vi "New Dashboard.vi"() -> ()   [LabVIEW 2015]
uses:
  <vilib>/Rock Robotics/Network Tables/NT Read Number.vi
  <vilib>/Rock Robotics/Network Tables/NT Read Numeric Array.vi
panel:
  out "MotorChart L":T1(graph)
  out "MotorSliders L":T2 {"MotorSlide4 2" scale=0.0..14.0 scale format="%#_2e"; "MotorSlide2" scale=-1.0..1.0 scale format="%#_2e"; "MotorSlide1" scale=-1.0..1.0 scale format="%#_2e"}
  out "MotorChart R":cluster{"Numeric":dbl, "Numeric":dbl}(graph)
  out "MotorSliders R":cluster{"MotorSlide1":dbl, "MotorSlide2":dbl} {"MotorSlide2" scale=-1.0..1.0 scale format="%#_2e"; "MotorSlide1" scale=-1.0..1.0 scale format="%#_2e"}
  out "JS1 Graph":cluster{"X":dbl, "Y":dbl}[](graph)
  out "JS1 Z":dbl(slide) scale=-1.0..1.0 scale format="%#_2e"
  out "JS1 Buttons":T3
  out "Gyro":dbl(knob) scale=0.0..360.0
  out "JS2 Graph":cluster{"X":dbl, "Y":dbl}[](graph)
  out "JS2 Z":dbl(slide) scale=-1.0..1.0 scale format="%#_2e"
  out "JS2 Buttons":T3
  out "Camera IP":string
  in  "TCP":refnum<k5>
  out "Mode":T4(ring)=enum."Auto Disabled"
  in  "Vision":u16(ring) items=["Camera Off", "USB Camera SW", "USB Camera HW", "IP Camera"]
  in  "Rec Mode":enum32{"Stop", "Record", "Playback"}(radio)
  out "Air Pressure":dbl(knob) scale=0.0..150.0
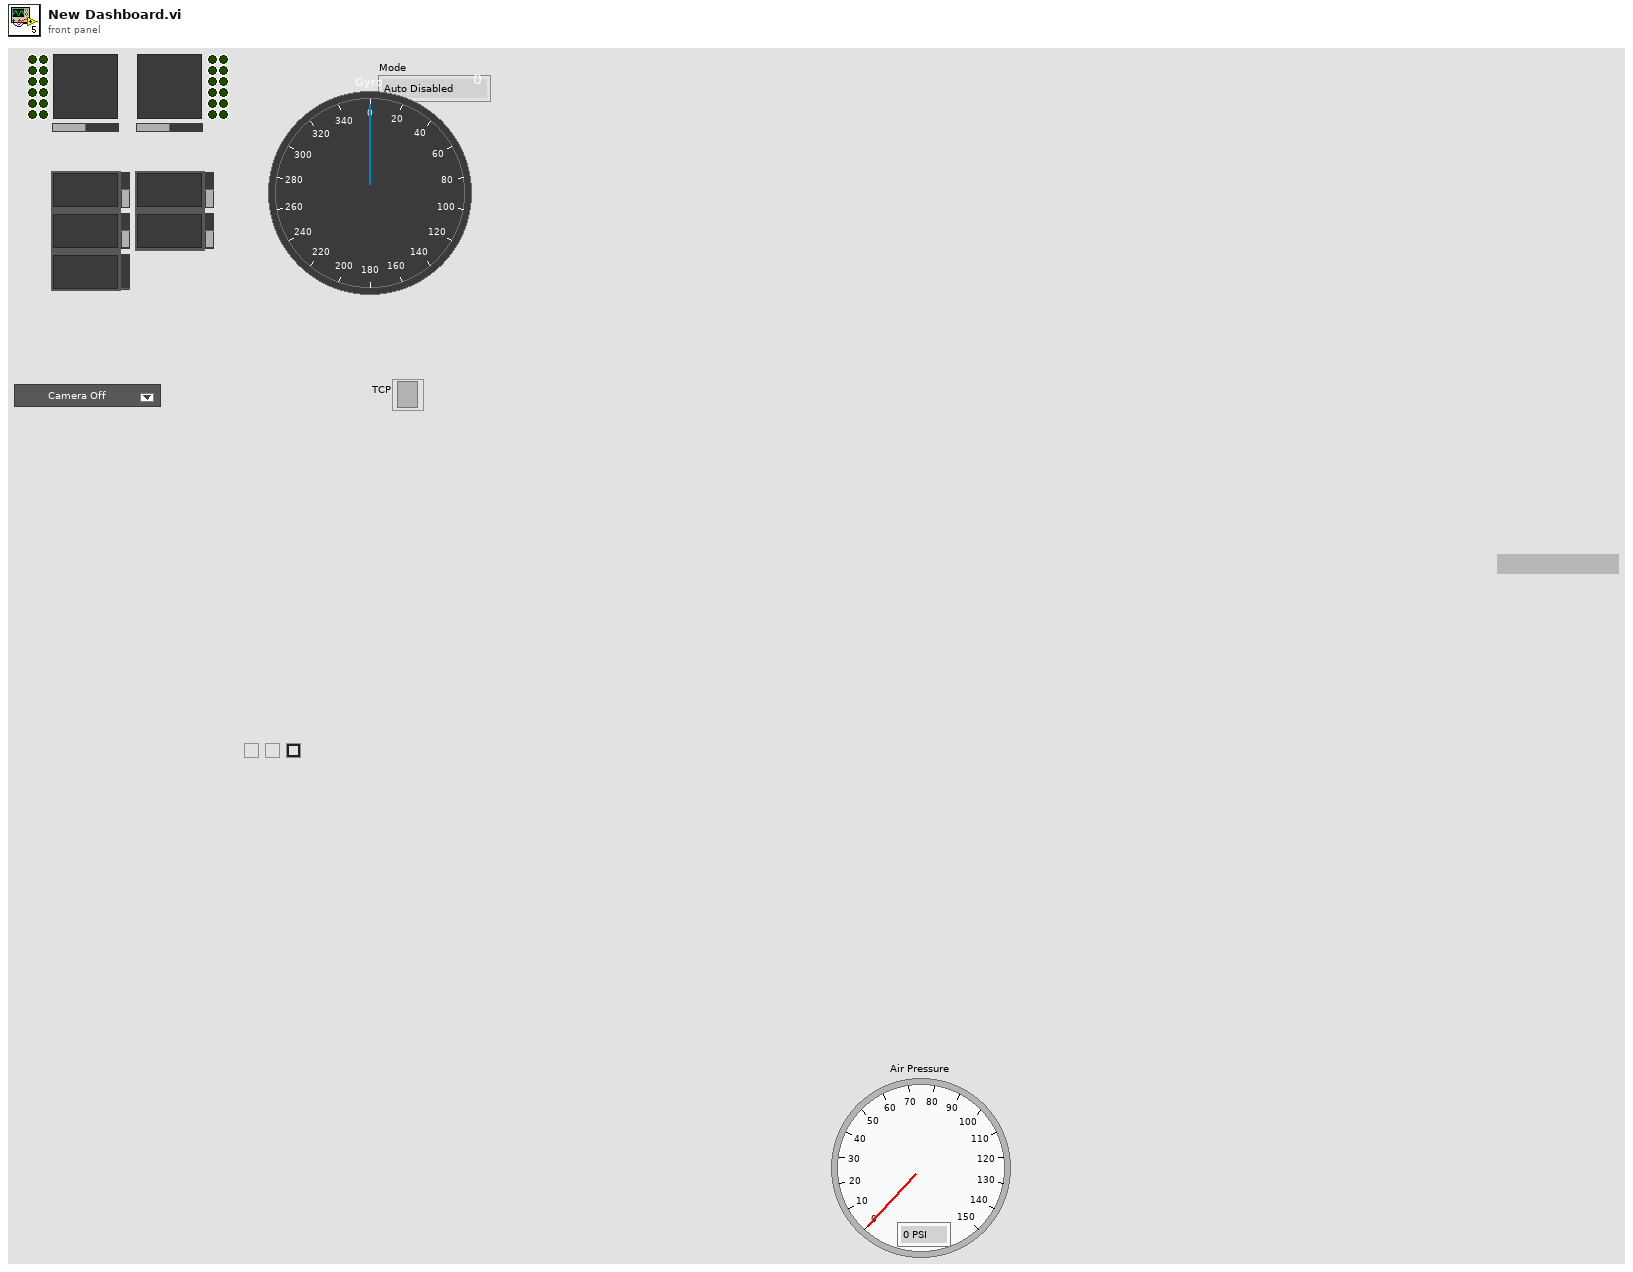
[diagram p1: front panel]
types:
  T1 = cluster{"Numeric":dbl, "Numeric":dbl, "Battery V":dbl}
  T2 = cluster{"MotorSlide1":dbl, "MotorSlide2":dbl, "MotorSlide4 2":dbl}
  T3 = cluster{bool, bool, bool, bool, bool, bool, bool, bool, bool, bool, bool, bool}
  T4 = enum8{"Tele-Op Disabled", "Tele-Op Enabled", "Auto Disabled", "Auto Enabled", "Test Disabled", "Test Enabled", "Disconnected", "No Code", "E-Stop"}
  T5 = cluster{"IDs":cluster{"RPC field ID":u16, "Unique ID":u16}, "String":string}
  T6 = cluster{"Error Strings":string, "Disable Counts":cluster{u16, u16}, "Rail Faults":cluster{u16, u16, u16}, "Robot IP":string, "DB Mode":u8, "Event Info":cluster{"Name":string, "Type":u8, "Number":u16, "Replay":u8}, "Camera Addr":string}
  T7 = cluster{"Storage":cluster{"Disk Free":u64, "RAM Block":u32, "RAM free":u32}, "CPU Utilization":cluster{"CPU % ISR":sgl, "CPU % Time Crit":sgl, "CPU % Timed Str":sgl, "CPU % High":sgl, "CPU % Above":sgl, "CPU % Normal":sgl, "CPU % Low":sgl}, "CAN":cluster{"% Bus Utilization":sgl, "Bus Off Cnt":u32, "TX_FIFO Full Cnt":u32, "Receive Error Cnt":u8, "Transmit Error Cnt":u8}, "HID":cluster{"HID Outputs":u32, "Rumble Low":u16, "Rumble High":u16}[]}
  T8 = cluster{"Status bits":cluster{"Test Mode":bool, "Autonomous":bool, "Enabled":bool, "Code Start":bool, "Brownout":bool, "Reserved 2":bool, "Reserved 3":bool, "E-Stop":bool}, "Code Trace":cluster{"Disabled":bool, "TeleOp":bool, "Auto":bool, "Test":bool}, "Controller Type":enum16{"unknown", "cRIO", "roboRio"}, "Code?":enum16{"unknown", "noCode", "code"}, "Battery V":dbl}
  T9 = cluster{"Control Bits":cluster{"TestMode":bool, "Autonomous":bool, "Enabled":bool, "FMS Present":bool, bool, bool, bool, "E-Stop":bool}, "Team Station ":u8, "Countdown":sgl, "Joystick Values":cluster{"Axes":dbl[], "Buttons":bool[], "POVs":i16[]}[]}
  T10 = cluster{"Axes":dbl[], "Buttons":bool[], "POVs":i16[]}[]
  T11 = cluster{"Axes":dbl[], "Buttons":bool[], "POVs":i16[]}
  T12 = cluster{"Buttons[0]":bool, "Buttons[1]":bool, "Buttons[2]":bool, "Buttons[3]":bool, "Buttons[4]":bool, "Buttons[5]":bool, "Buttons[6]":bool, "Buttons[7]":bool, "Buttons[8]":bool, "Buttons[9]":bool, "Buttons[10]":bool, "Buttons[11]":bool}
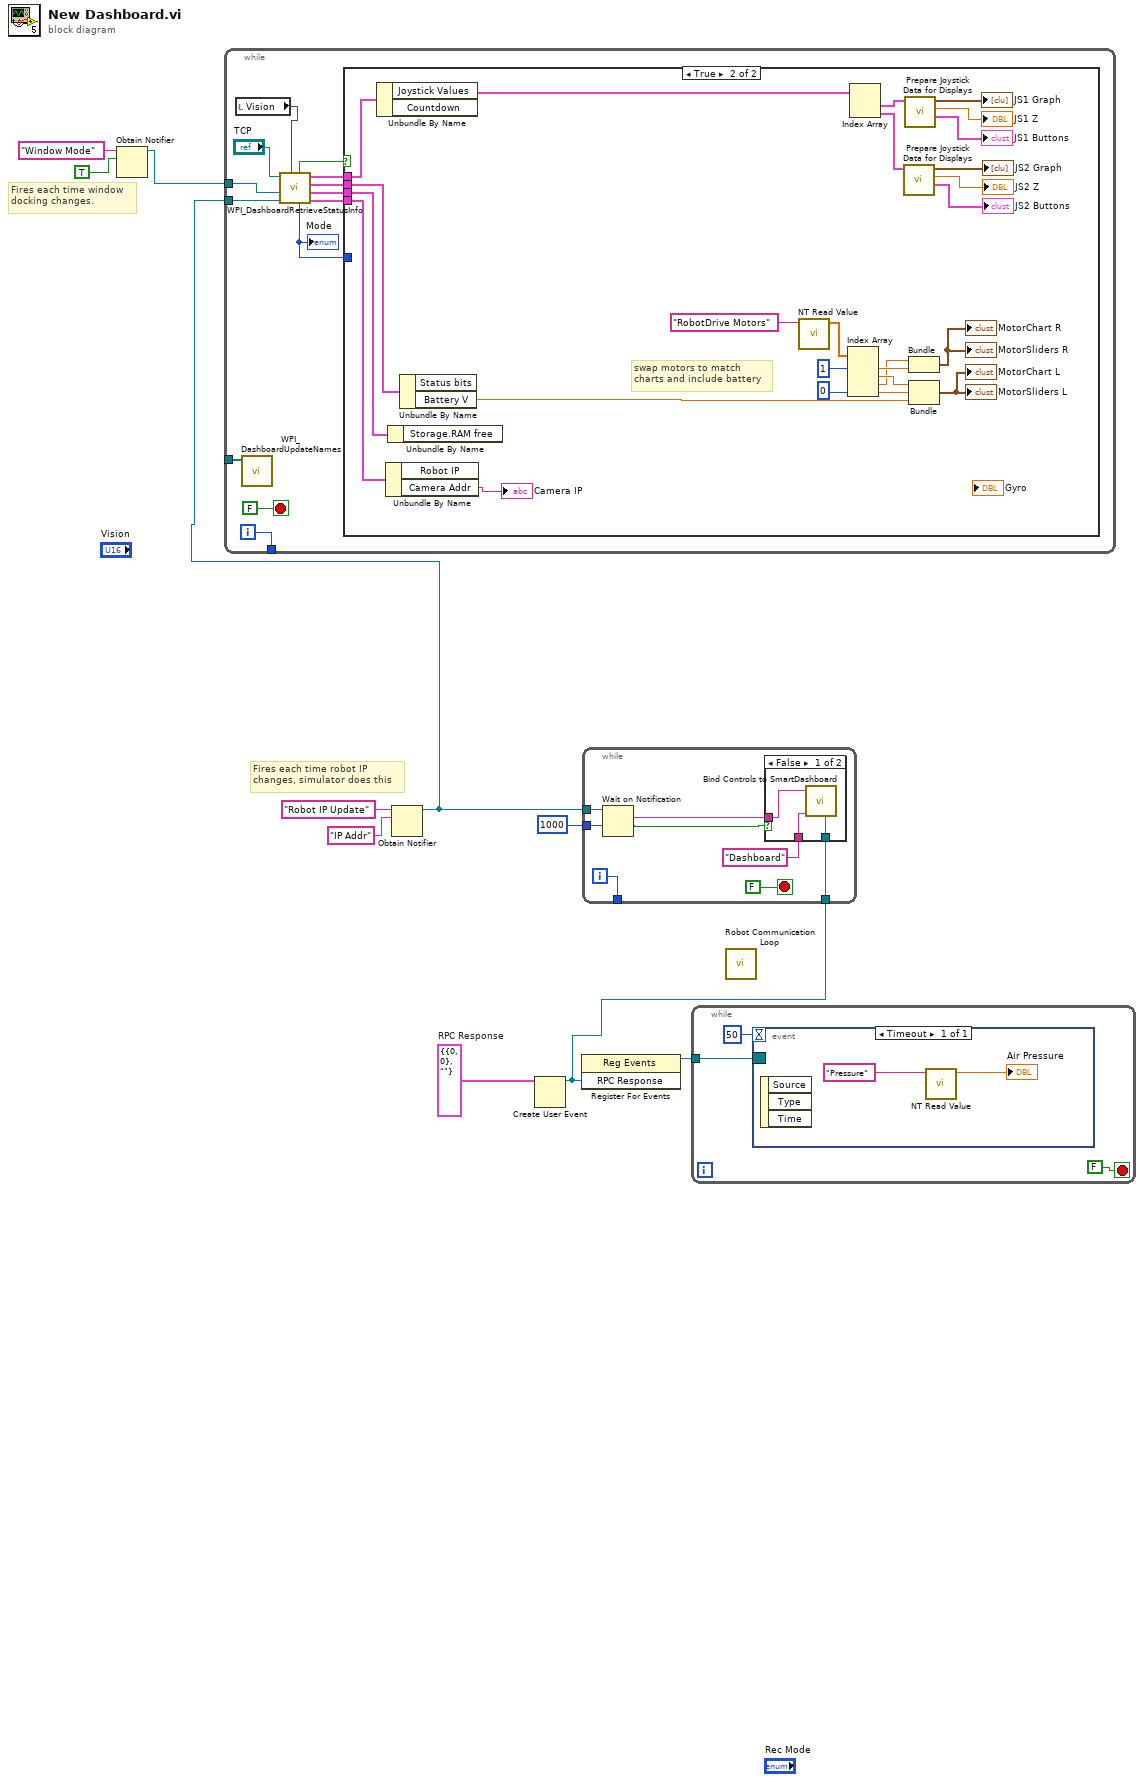
[diagram p0: block diagram]
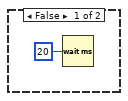
[diagram p2: hidden frame]
diagram:
  w10 = T5 {"IDs"={"RPC field ID"=0, "Unique ID"=0}, "String"=""}  # RPC Response
  # "Fires each time window\ndocking changes."
  # "Fires each time robot IP\nchanges, simulator does this"
  n1 = Obtain Notifier(name (unnamed)="Window Mode", notification data type=TRUE) -> (notifier out=w1:refnum<notifier>)  [unwired: 2 in, 2 out]
  n2 = Obtain Notifier(name (unnamed)="Robot IP Update", notification data type="IP Addr" ("name (unnamed)")) -> (notifier out=w4:refnum<notifier>)  [unwired: 2 in, 2 out]
  n3 = while {
    tunnel: [w22] -> _
    tunnel: _ -> [w16]
    tunnel: w4 -> [w12]
    tunnel: w1 -> [w11]
    i -> [w22]
    stop <- FALSE stop-if-true
    n4 = local read "Vision"() -> (w14:u16)
    n5 = call <vilib>:"WPI_DashboardUpdateNames.vi"("Controls on Tab"=w16) -> ()  [unwired: 11 in]
    n6 = call <vilib>:"WPI_DashboardRetrieveStatusInfo.vi"("Vision"=w14, "Binding Refnum"=w12, "Window Mode Notifier"=w11, "TCP Cnx"="TCP") -> ("Power and Errors"=w17:T6, "Robot Metrics"=w20:T7, "Status Info"=w21:T8, "Control Info"=w18:T9, "Robot Mode"=w15:T4, "Process?"=w19:bool)  [unwired: 2 in]
    "Mode" <- w15
    n7 = case shown="True" w19 {
      tunnel: w21 -> [_ w49]
      tunnel: w20 -> [_ w48]
      tunnel: w18 -> [_ w47]
      tunnel: w17 -> [_ w46]
      tunnel: w15 -> [_ _]
      frame False {
        n8 = Wait (ms)(milliseconds to wait=u32 20) -> ()  [unwired: 1 out]
      }
      frame True {
        # "swap motors to match\ncharts and include battery"
        n9 = Unbundle By Name(w47) -> ("Joystick Values"=w36:T10)  [unwired: 1 out]
        n10 = Unbundle By Name(w46) -> ("Camera Addr"=→"Camera IP":string)  [unwired: 1 out]
        n11 = Unbundle By Name(w48) -> ()  [unwired: 1 out]
        n12 = Unbundle By Name(w49) -> ("Battery V"=w37:dbl)  [unwired: 1 out]
        n13 = call-poly <vilib>:"NT Read Value.vi"("Name"="RobotDrive Motors") -> ("Numeric Array"=w25:dbl[])  [unwired: 9 in, 1 out]
        n14 = Index Array(array=w25, index #1=1, index #4=0) -> (element #1=w41:dbl, element #2=w42:dbl, element #3=w40:dbl, element #4=w45:dbl)  [unwired: 2 in]
        n15 = Index Array(array=w36) -> (element #1=w35:T11, element #2=w30:T11)  [unwired: 2 in]
        n16 = call "Prepare Joystick Data for Displays.vi"("Joystick Values"=w30) -> ("Buttons"=→"JS2 Buttons":T12, "Z Axis"=→"JS2 Z":dbl, "Cartesian Data"=→"JS2 Graph":cluster{"X axis":dbl, "X axis":dbl}[])  [unwired: 8 in]
        n17 = call "Prepare Joystick Data for Displays.vi"("Joystick Values"=w35) -> ("Buttons"=→"JS1 Buttons":T12, "Z Axis"=→"JS1 Z":dbl, "Cartesian Data"=→"JS1 Graph":cluster{"X axis":dbl, "X axis":dbl}[])  [unwired: 8 in]
        n18 = Bundle("Numeric"=w40, "Numeric"=w41) -> (→"MotorChart R" →"MotorSliders R":cluster{"Numeric":dbl, "Numeric":dbl})  [unwired: 1 in]
        n19 = Bundle("Numeric"=w42, "Numeric"=w45, "Battery V"=w37) -> (→"MotorChart L" →"MotorSliders L":T1)  [unwired: 1 in]
      }
    }
  }
  n20 = Create User Event(user event datatype=w10) -> (user event=w5:refnum<user-event>)  [unwired: 1 in, 1 out]
  n21 = register-events(w5) -> (reference out=w9:refnum<event-registration>)  [unwired: 2 in, 1 out]
  n22 = while {
    tunnel: w4 -> [w56]
    tunnel: [w54] -> _
    tunnel: w5 -> [w52]
    tunnel: u32 1000 ("milliseconds to wait") -> [w51]
    i -> [w54]
    stop <- FALSE stop-if-true
    n23 = Wait on Notification(notifier=w56, timeout in ms (-1)=w51) -> (notification=w55:string, timed out?=w50:bool)  [unwired: 2 in, 2 out]
    n24 = case shown="False" w50 {
      tunnel: w55 -> [w60 _]
      tunnel: "Dashboard" -> [w59 _]
      tunnel: w52 -> [w58 _]
      frame False {
        n25 = call <vilib>:"Bind Controls to SmartDashboard.vi"("RPC ref"=w58, "Client Name"=w59, "Server IP Address"=w60) -> ()  [unwired: 9 in]
      }
      frame True {
      }
    }
  }
  n26 = while {
    tunnel: w9 -> [w62]
    stop <- FALSE stop-if-true
    n27 = event shown="[0] Timeout" {
      selector: w62 -> [_]
      dyn-events: _ -> [_]
      timeout: 50 -> [_]
      event Timeout {
        n28 = event-data() -> ()  [unwired: 1 in, 3 out]
        n29 = call-poly <vilib>:"NT Read Value.vi"("Name"="Pressure") -> ("Numeric"=→"Air Pressure":dbl)  [unwired: 9 in, 1 out]
      }
    }
  }
  n30 = call "Robot Communication Loop.vi"() -> ()  [unwired: 12 in]
